vi "Create_DO_Signal.vi"(8 "error in":errorcluster, 10 "Pre-Activation?":bool, 11 "On/Off":bool) -> (0 "error out":errorcluster, 2 "Samples":u32, 3 "WF":u8[](array[numeric]))   [LabVIEW 2025]
panel:
  out "Waveform Graph":u32[](graph)
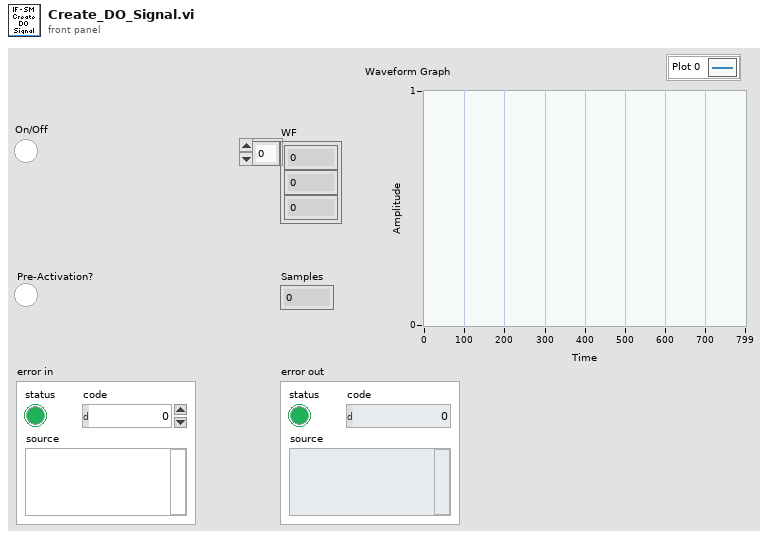
[diagram p1: front panel]
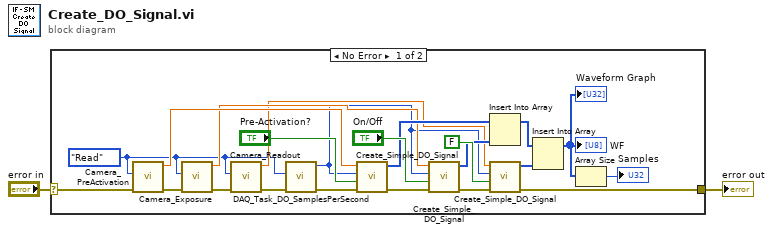
[diagram p0: block diagram]
diagram:
  n1 = case shown="No Error" "error in" {
    selector: "error in" -> [w13 w25]
    tunnel: [w5 w25] -> w1
    frame No Error {
      w3 = enum16{"Init", "Write", "Read"}."Read" ("Action")
      n2 = call "Camera_PreActivation.vi"("error in"=w13, "Action"=w3) -> ("error out"=w12:errorcluster, "Camera_PreActivation"=w14:dbl)  [unwired: 8 in]
      n3 = call "Camera_Exposure.vi"("error in"=w12, "Action"=w3) -> ("error out"=w10:errorcluster, "Exposure (s)"=w11:dbl)  [unwired: 8 in]
      n4 = call "Camera_Readout.vi"("error in"=w10, "Action"=w3) -> ("error out"=w8:errorcluster, "Camera_Readout"=w9:dbl)  [unwired: 8 in]
      n5 = call "DAQ_Task_DO_SamplesPerSecond.vi"("error in"=w8, "Action"=w3) -> ("error out"=w6:errorcluster, "DO_Task_SamplesPerSec"=w7:u32)  [unwired: 8 in]
      n6 = call "Create_Simple_DO_Signal.vi"("error in"=w6, "On/Off"="Pre-Activation?", "Samples / s (10000)"=w7, "Time (s)"=w14) -> ("error out"=w17:errorcluster, "Signal"=w15:u32[])  [unwired: 6 in]
      n7 = call "Create_Simple_DO_Signal.vi"("error in"=w17, "On/Off"="On/Off", "Samples / s (10000)"=w7, "Time (s)"=w11) -> ("error out"=w19:errorcluster, "Signal"=w18:u32[])  [unwired: 6 in]
      n8 = Insert Into Array(array=w15, new element=w18) -> (w20:u32[])  [unwired: 1 in]
      n9 = call "Create_Simple_DO_Signal.vi"("error in"=w19, "On/Off"=FALSE, "Samples / s (10000)"=w7, "Time (s)"=w9) -> ("error out"=w5:errorcluster, "Signal"=w21:u32[])  [unwired: 6 in]
      n10 = Insert Into Array(array=w20, new element=w21) -> (w4:u32[])  [unwired: 1 in]
      "WF" <- w4
      "Waveform Graph" <- w4
      n11 = Array Size(array=w4) -> (size(s)=→"Samples":i32)
    }
    frame Error {
    }
  }
  "error out" <- w1
